vi "FGPA Main for MAX5216.vi"() -> ()   [LabVIEW 2015]
doc: "This is the main FPGA VI for the SPI application. It sets up the SPI communication and then runs the SPI engine. In a parallel loop, data is continually read from the Real Time application and sent to the SPI engine. The SPI engine handles all communication between the FPGA and the SPI chip."
uses:
  <userlib>/_NI SPI IP/FPGA/Controllers/Public/Transfer Settings.ctl
  vi.lib/SPIAPI/Controls/SPI API DIO Enable Lines.ctl
  <vilib>/Platform/TimedLoop/XDataNode/timing_clust.ctl
  <vilib>/Platform/TimedLoop/XDataNode/nitl_modes.ctl
  <vilib>/Platform/TimedLoop/XDataNode/wakeup.ctl
  vi.lib/SPIAPI/Controls/SPI API DIO Lines.ctl
  <vilib>/rvi/Emulation/niFpgaGetClockAttributes.vi
  <vilib>/rvi/Emulation/niFpgaSctlEmulationGetInTimedLoop.vi
  <vilib>/rvi/Emulation/niFpgaEmulationReportErrorSimple.vi
  <vilib>/rvi/Emulation/niFpgaCriticalErrorInLSC.vi
  <vilib>/Platform/TimedLoop/XDataNode/XDataNode.xnode
  <vilib>/Platform/TimedLoop/XDataNode/XDNodeRunTimeDep.lvlib
  <userlib>/_NI SPI IP/FPGA/Controllers/NI SPI IP FPGA.lvlib
panel:
  out "Slave Response":u64
  out "read Iterations":i32
  in  "Data To DAC":u64=2147483648
  in  "Chip Select":u8
  in  "SPI Physical Settings":T1={"Divide Value"=20, "Transfer Length (bits)"=32, "CS Asserted Polarity"=FALSE, "Clock Polarity (CPOL)"=FALSE, "Clock Phase (CPHA)"=FALSE, "Lengthen MISO Setup"=FALSE, "Direction Change Bit"=0, "MOSI Starts as Output"=FALSE, "Tristatable MOSI"=FALSE} {"Direction Change Bit" max=64 step=1; "Transfer Length (bits)" min=1 max=64 step=1}
  in  "Sample Rate (S/s)":u32=10000
  out "oclk freq":u32
  out "oclk div":u32
  out "FPGA Error":errorcluster
  out "Actual Loop Ticks":u32
  # "Overview: This is the FPGA VI that communicates with the MAX5216.\nRequirements: LabVIEW Full Development System, LabVIEW Real Time,  LabVIEW FPGA, MAX5216, NI System on Module, NI 9651.\nInstructions:\nRun RT Main without making adjustments to this VI to avoid a recompile.  If you desire to adjust this VI, do so, \nthen be sure to point RT Main to this VI instead of the pre-compiled bitfile that it currently targets."
  # "OUTPUT"
  # "INPUT"
  # "ADC Data::Debug"
  # "Acquisition Parameters"
  # "SPI Settings"
  # "Debug"
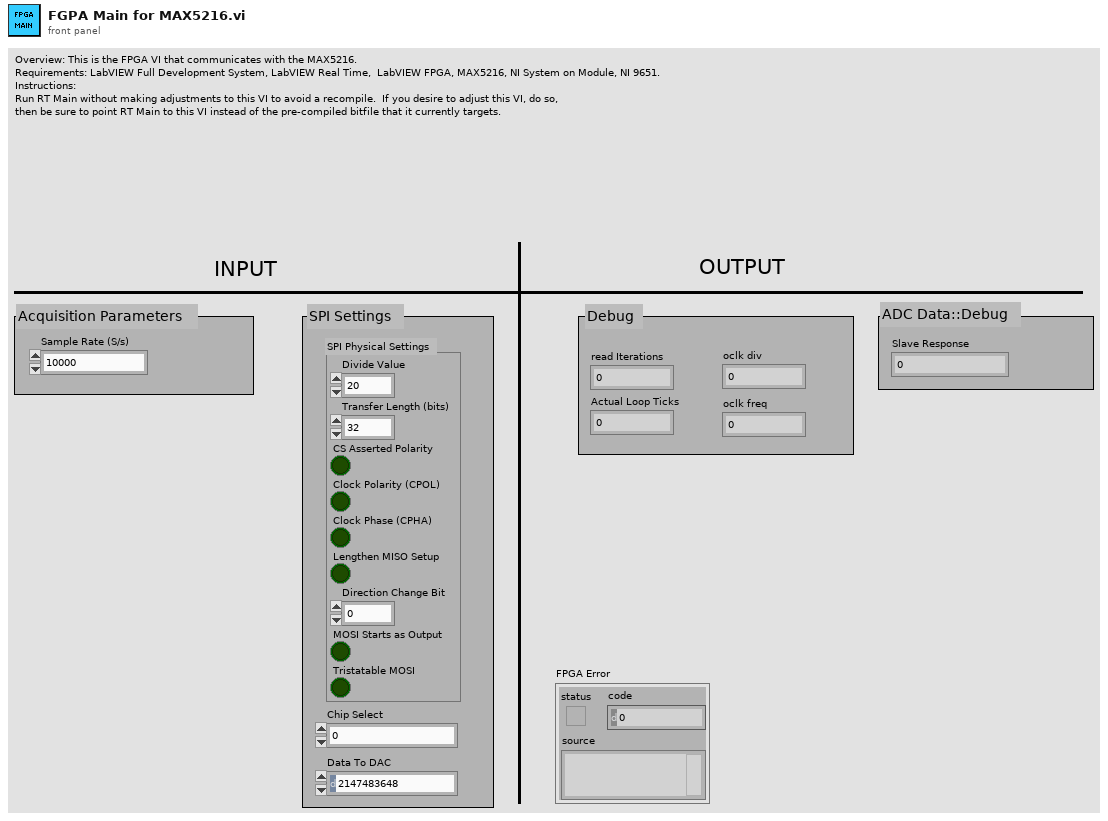
[diagram p1: front panel]
types:
  T1 = typedef "NI SPI IP FPGA.lvlib/Transfer Settings.ctl" = cluster{"Divide Value":u8, "Transfer Length (bits)":u8, "CS Asserted Polarity":bool, "Clock Polarity (CPOL)":bool, "Clock Phase (CPHA)":bool, "Lengthen MISO Setup":bool, "Direction Change Bit":u8, "MOSI Starts as Output":bool, "Tristatable MOSI":bool}
  T2 = typedef "SPI API DIO Lines.ctl" = cluster{"SCLK":refnum<k21>, "MISO":refnum<k21>, "MOSI":refnum<k21>, "CS 0":refnum<k21>, "CS 1":refnum<k21>, "CS 2":refnum<k21>, "CS 3":refnum<k21>, "CS 4":refnum<k21>, "CS 5":refnum<k21>}
  T3 = typedef "SPI API DIO Enable Lines.ctl" = cluster{"SCLK_en":refnum<k21>, "MISO_en":refnum<k21>, "MOSI_en":refnum<k21>, "CS0_en":refnum<k21>, "CS1_en":refnum<k21>, "CS2_en":refnum<k21>, "CS3_en":refnum<k21>, "CS4_en":refnum<k21>, "CS5_en":refnum<k21>}
  T4 = typedef "SPI API References.ctl" = cluster{"DLU To SPI Engine Data FIFO":refnum<k21>, "SPI Engine to DLU Data FIFO":refnum<k21>, "Data to SPI Engine (Cache) Register":refnum<k21>, "SPI Settings to SPI Engine (Cache) Register":refnum<k21>}
  T5 = typedef "XDNodeRunTimeDep.lvlib/timing_clust.ctl" = cluster{"Expected End [f-1]":u64, "Actual End [f-1]":u64, "Finished Late? [f-1]":bool, "Expected End [i-1]":u64, "Actual End [i-1]":u64, "Finished Late? [i-1]":bool, "Expected Start [i]":u64, "Actual Start [i]":u64, "Expected Start [f]":u64, "Actual Start [f]":u64, "Source Name":string, "Structure Name":string, "Period":i64, "Deadline":i64, "Offset":i64, "Start":i64, "Priority":i32, "Timeout":i32, "Mode":T6, "Wakeup Reason":T7, "Error":errorcluster, "Source Type":string, "Secondary Source Type":string, "Global End Time":u64, "Global Start Time":u64, "Frame Duration":u64, "Iteration Duration":u64, "Assigned CPU":i32, "I/O Scan Engine Mode":u32}
  T6 = typedef "XDNodeRunTimeDep.lvlib/nitl_modes.ctl" = enum32{"No Change", "Process missed periods, maintain original phase", "Discard missed periods, maintain original phase", "Process missed periods, ignore original phase", "Discard missed periods, ignore original phase"}
  T7 = typedef "XDNodeRunTimeDep.lvlib/wakeup.ctl" = enum32{"Normal", "Aborted", "Asynchronous wakeup", "Timing source error", "Timed loop error", "Timeout"}
  T8 = typedef "SPI API Response Data.ctl" = cluster{"Data to Node":u64, "Node Id":u16}
  T9 = typedef "NI SPI IP FPGA.lvlib/Spi Master Inputs.ctl" = cluster{"MISO":bool}
  T10 = typedef "NI SPI IP FPGA.lvlib/Spi Master Outputs.ctl" = cluster{"Chip Select":bool, "Clock":bool, "MOSI":bool, "MOSI OE":bool}
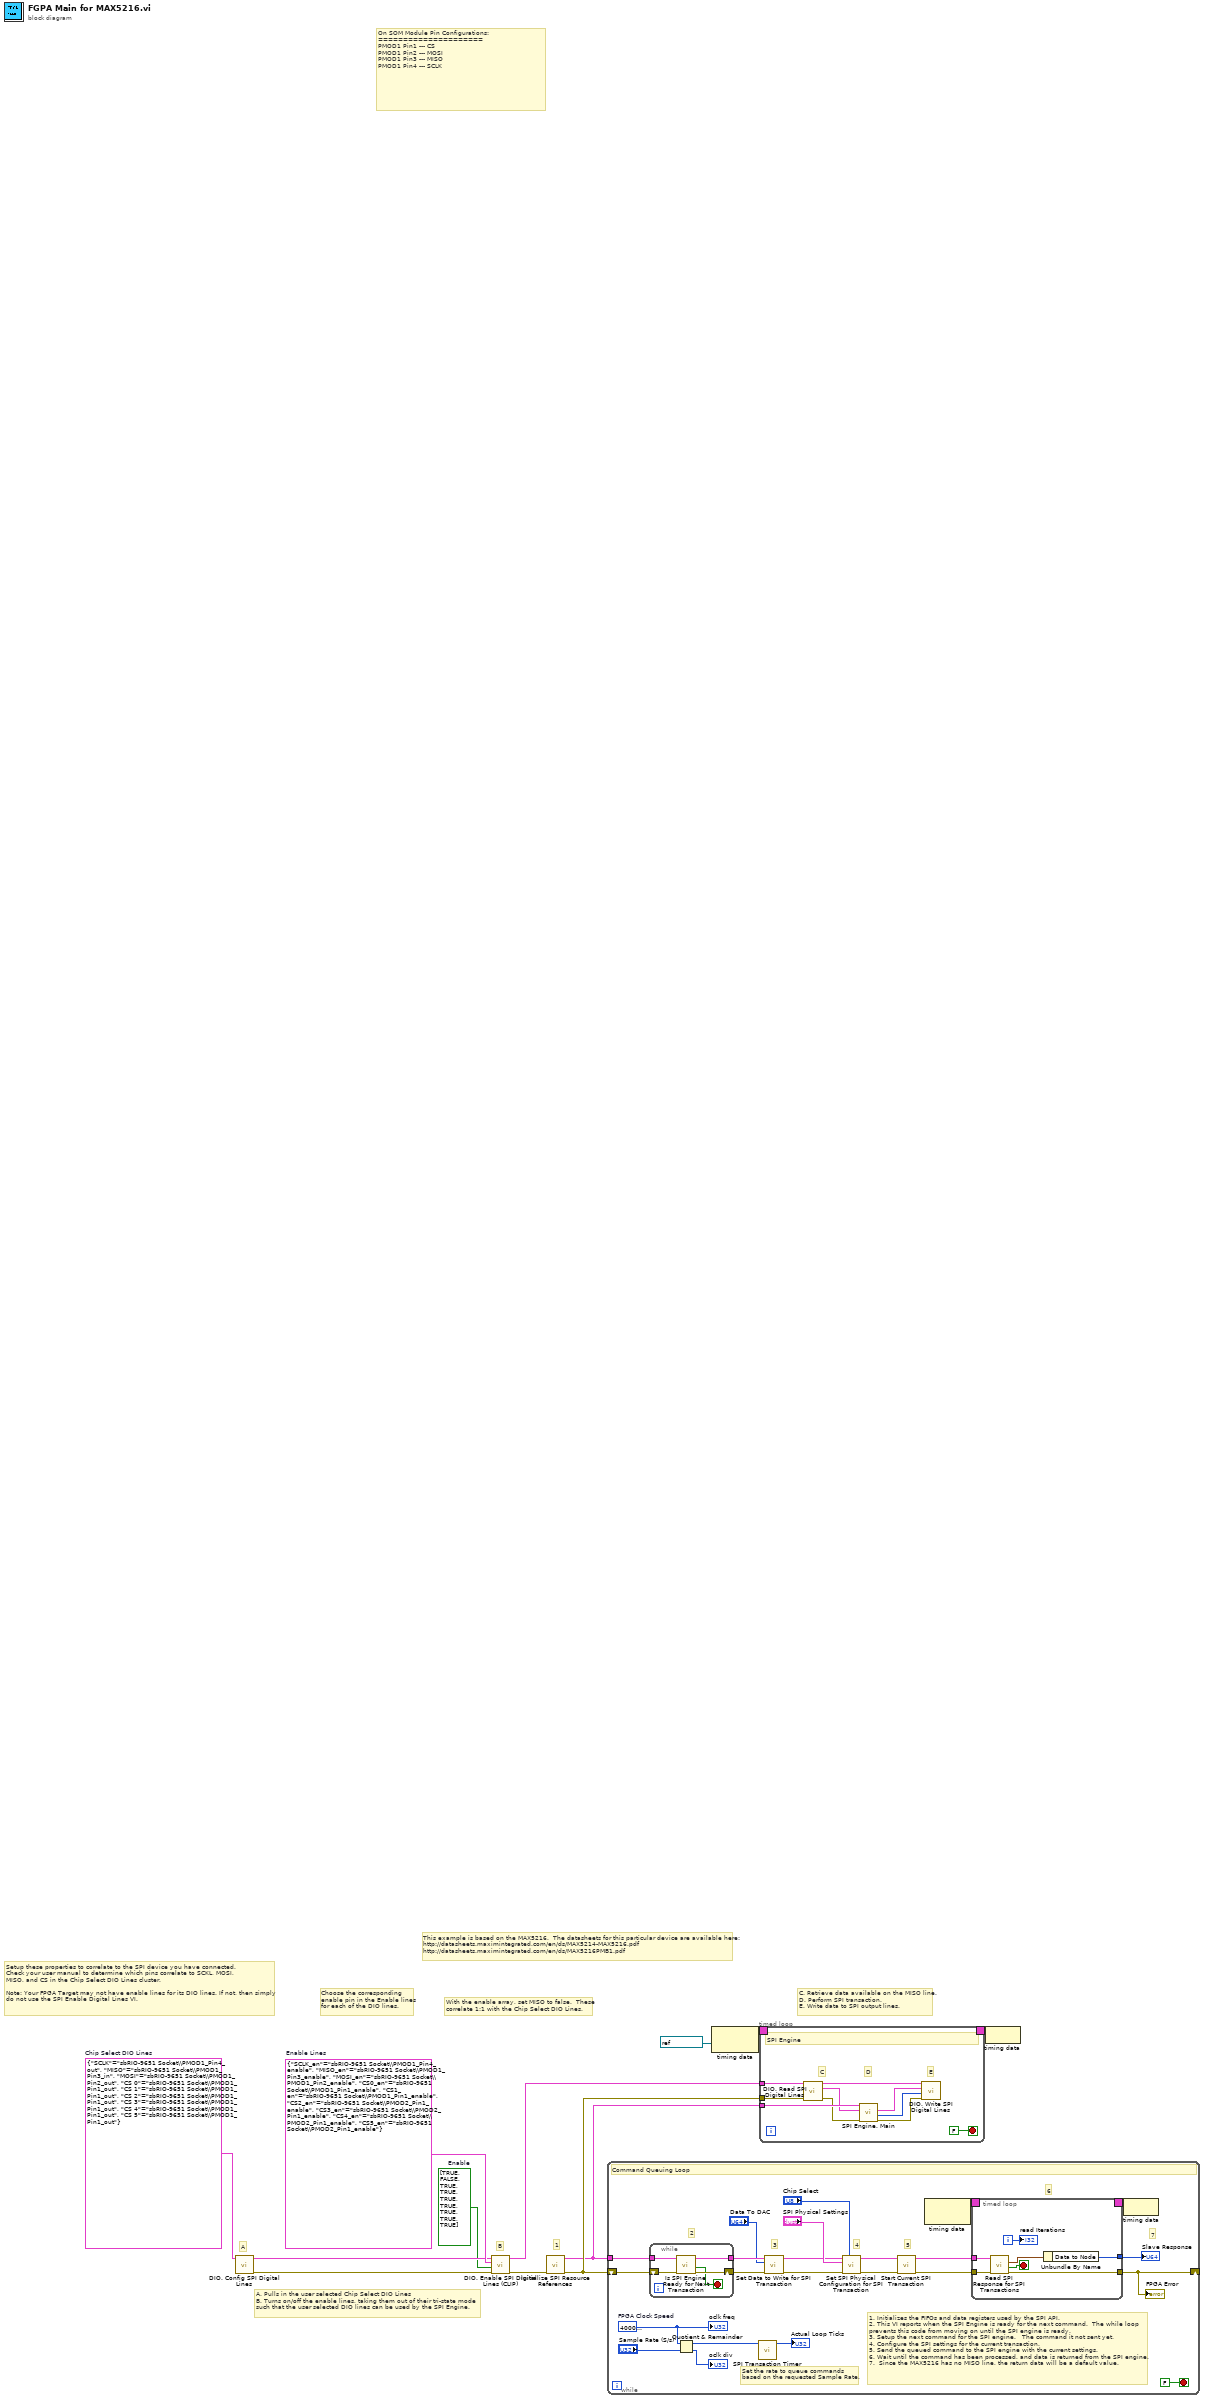
[diagram p0: block diagram]
diagram:
  w5 = T2 {"SCLK"="sbRIO-9651 Socket\\PMOD1_Pin4_out", "MISO"="sbRIO-9651 Socket\\PMOD1_Pin3_in", "MOSI"="sbRIO-9651 Socket\\PMOD1_Pin2_out", "CS 0"="sbRIO-9651 Socket\\PMOD1_Pin1_out", "CS 1"="sbRIO-9651 Socket\\PMOD1_Pin1_out", "CS 2"="sbRIO-9651 Socket\\PMOD1_Pin1_out", "CS 3"="sbRIO-9651 Socket\\PMOD1_Pin1_out", "CS 4"="sbRIO-9651 Socket\\PMOD1_Pin1_out", "CS 5"="sbRIO-9651 Socket\\PMOD1_Pin1_out"}  # Chip Select DIO Lines
  w4 = bool[] [TRUE, FALSE, TRUE, TRUE, TRUE, TRUE, TRUE, TRUE, TRUE]  # Enable
  w12 = T3 {"SCLK_en"="sbRIO-9651 Socket\\PMOD1_Pin4_enable", "MISO_en"="sbRIO-9651 Socket\\PMOD1_Pin3_enable", "MOSI_en"="sbRIO-9651 Socket\\PMOD1_Pin2_enable", "CS0_en"="sbRIO-9651 Socket\\PMOD1_Pin1_enable", "CS1_en"="sbRIO-9651 Socket\\PMOD1_Pin1_enable", "CS2_en"="sbRIO-9651 Socket\\PMOD2_Pin1_enable", "CS3_en"="sbRIO-9651 Socket\\PMOD2_Pin1_enable", "CS4_en"="sbRIO-9651 Socket\\PMOD2_Pin1_enable", "CS5_en"="sbRIO-9651 Socket\\PMOD2_Pin1_enable"}  # Enable Lines
  # "Choose the corresponding\nenable pin in the Enable lines\nfor each of the DIO lines."
  # "With the enable array, set MISO to false.  These\ncorrelate 1:1 with the Chip Select DIO Lines."
  # "A. Pulls in the user selected Chip Select DIO Lines\nB. Turns on/off the enable lines, taking them out of their tri-state mode \nsuch that the user selected DIO lines can be used by the SPI Engine."
  # "This example is based on the MAX5216.  The datasheets for this particular device are available here:\nhttp://datasheets.maximintegrated.com/en/ds/MAX5214-MAX5216.pdf\nhttp://datasheets.maximintegrated.com/en/ds/MAX5216PMB1.pdf"
  # "C. Retrieve data available on the MISO line.\nD. Perform SPI transaction.\nE. Write data to SPI output lines."
  # "B"
  # "A"
  # "1"
  # "Setup these properties to correlate to the SPI device you have connected.\nCheck your user manual to determine which pins correlate to SCKL, MOSI,\nMISO, and CS in the Chip Select DIO Lines cluster.\n\nNote: Your FPGA Target may not have enable lines for its DIO lines. If not, then simply\ndo not use the SPI Enable Digital Lines VI."
  # "On SOM Module Pin Configurations:\n=====================\nPMOD1 Pin1 --- CS\nPMOD1 Pin2 --- MOSI\nPMOD1 Pin3 --- MISO\nPMOD1 Pin4 --- SCLK"
  n1 = call "DIO. Config SPI Digital Lines.vi"("SPI DIO Lines"=w5) -> ("error out"=w6:errorcluster, "Chip Select DIO Lines"=w7:T2)  [unwired: 9 in]
  n2 = call "DIO. Enable SPI Digital Lines (CLIP).vi"("error in"=w6, "Enable"=w4, "Enable Lines"=w12, "SPI DIO Lines"=w7) -> ("error out"=w3:errorcluster, "Chip Select DIO Lines"=w8:T2)  [unwired: 6 in]
  n3 = call "Initialize SPI Resource References.vi"("error in"=w3) -> ("error out"=w2:errorcluster, "SPI API References"=w1:T4)  [unwired: 9 in]
  n4 = while {
    shift-right: [w14] -> _
    shift-left: w2 -> [w31]
    tunnel: w1 -> [w32]
    stop <- FALSE stop-if-true
    w18 = u32 40000000  # FPGA Clock Speed
    # "1. Initializes the FIFOs and data registers used by the SPI API.\n2. This VI reports when the SPI Engine is ready for the next command.  The while loop \nprevents this code from moving on until the SPI engine is ready.\n3. Setup the next command for the SPI engine.   The command it not sent yet.\n4. Configure the SPI settings for the current transaction.\n5. Send the queued command to the SPI engine with the current settings.\n6. Wait until the command has been processed, and data is returned from the SPI engine.\n7.  Since the MAX5216 has no MISO line, the return data will be a default value."
    # "Set the rate to queue commands\nbased on the requested Sample Rate."
    # "7"
    # "6"
    # "5"
    # "4"
    # "3"
    # "2"
    # "Command Queuing Loop"
    n5 = while {
      shift-right: [w40] -> w34
      shift-left: w31 -> [w37]
      tunnel: w32 -> [w38]
      tunnel: [w39] -> w33
      stop <- w36 stop-if-true
      n6 = call "Is SPI Engine Ready for Next Transaction.vi"("error in"=w37, "Private Data In"=w38) -> ("error out"=w40:errorcluster, "SPI Channel Ready"=w36:bool, "Private Data Out"=w39:T4)  [unwired: 6 in, 1 out]
    }
    n7 = Quotient & Remainder(x=w18, y="Sample Rate (S/s)") -> (x-y*floor(x/y)=w15:u32, floor(x/y)=→"oclk div":u32)
    n8 = call "SPI Transaction Timer.vi"("Loop Time (Ticks)"=w15) -> ("Actual Time (Ticks)"=→"Actual Loop Ticks":u32)  [unwired: 10 in]
    n9 = call "Set Data to Write for SPI Transaction.vi"("error in"=w34, "Data In"="Data To DAC", "Private Data In"=w33) -> ("error out"=w25:errorcluster, "Private Data Out"=w26:T4)  [unwired: 7 in]
    n10 = call "Set SPI Physical Configuration for SPI Transaction.vi"("Chip Select"="Chip Select", "error in"=w25, "SPI Physical Settings"="SPI Physical Settings", "Private Data In"=w26) -> ("error out"=w22:errorcluster, "Private Data Out"=w23:T4)  [unwired: 6 in]
    n11 = call "Start Current SPI Transaction.vi"("error in"=w22, "Private Data In"=w23) -> ("error out"=w27:errorcluster, "Private Data Out"=w21:T4)  [unwired: 7 in, 1 out]
    n12 = node-c288() -> (w30:T5)  [unwired: 1 in]
    n13 = timed-loop {
      timing: w30 -> [_]
      timing-out: [_] -> w29
      tunnel: w27 -> [w47]
      tunnel: w21 -> [w46]
      tunnel: [w41] -> w19
      tunnel: [w43] -> w14
      i -> [w42]
      stop <- w45 stop-if-true
      n14 = call "Read SPI Response for SPI Transactions.vi"("error in"=w47, "Private Data In"=w46) -> ("error out"=w43:errorcluster, "Read Data Valid?"=w45:bool, "Read Data"=w44:T8)  [unwired: 6 in, 1 out]
      n15 = Unbundle By Name(w44) -> ("Data to Node"=w41:u64)
      "read Iterations" <- w42
    }
    "Slave Response" <- w19
    "FPGA Error" <- w14
    n16 = node-c288(w29) -> ()
    "oclk freq" <- w18
  }
  n17 = node-c288(refnum<k21> "120MHz" ("Source Name")) -> (w11:T5)
  n18 = timed-loop {
    tunnel: w1 -> [w58]
    tunnel: w2 -> [w56]
    tunnel: w8 -> [w60]
    timing: w11 -> [_]
    timing-out: [_] -> w10
    stop <- FALSE stop-if-true
    # "E"
    # "D"
    # "C"
    # "SPI Engine"
    n19 = call "DIO. Read SPI Digital Lines.vi"("Chip Select DIO Lines"=w60, "error in"=w56) -> ("Chip Select DIO Lines Out"=w61:T2, "SPI Read Data"=w57:T9, "error out"=w55:errorcluster)  [unwired: 11 in]
    n20 = call "SPI Engine. Main.vi"("error in"=w55, "SPI Read Data"=w57, "SPI API References"=w58) -> ("error out"=w54:errorcluster, "Chip Select ID"=w53:u8, "SPI DIO Output"=w59:T10)  [unwired: 5 in, 1 out]
    n21 = call "DIO. Write SPI Digital Lines.vi"("error in"=w54, "CS Index"=w53, "spi output"=w59, "Chip Select DIO Lines"=w61) -> ()  [unwired: 6 in, 2 out]
  }
  n22 = node-c288(w10) -> ()
